vi "SLSC Parse Path String.vi"(8 "error in (no error)":errorcluster, 11 "SLSC Channel Path":string) -> (0 "error out":errorcluster, 1 "Property or Command":string, 2 "Physical Channel":string, 3 "Datatype":string)   [LabVIEW 2020, in "SLSC CD Shared.lvlib"]
uses:
  SLSC CD Shared.lvlib
  <vilib>/regexp/Match Regular Expression.xnode
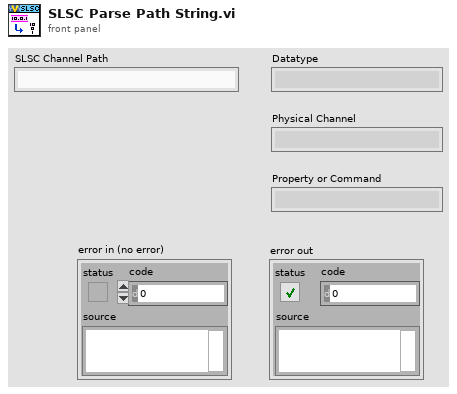
[diagram p1: front panel]
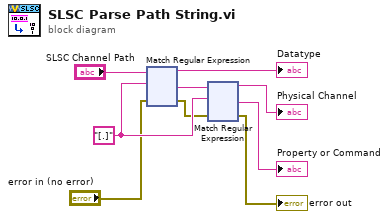
[diagram p0: block diagram]
diagram:
  w5 = "[.]" ("regular expression")
  n1 = xnode "Match Regular Expression"("input string"="SLSC Channel Path", "regular expression"=w5, "error in"="error in (no error)") -> ("before match"=→"Datatype":string, "after match"=w8:string, "error out"=w2:errorcluster)  [unwired: 3 in, 2 out]
  n2 = xnode "Match Regular Expression"("input string"=w8, "regular expression"=w5, "error in"=w2) -> ("before match"=→"Physical Channel":string, "after match"=→"Property or Command":string, "error out"=→"error out":errorcluster)  [unwired: 3 in, 2 out]
